vi "PLC Struct Byte Stream to G Object.vi"(8 "error in (no error)":errorcluster, 9 "[Sub-Item Type Information]":T1[](array[typedef]), 10 "Byte Stream":u8[](array[numeric]), 11 "TwinCAT ADS in":refnum<class "TwinCAT ADS.lvclass">) -> (0 "error out":errorcluster, 2 "Value":variant, 3 "TwinCAT ADS out":refnum<class "TwinCAT ADS.lvclass">)   [LabVIEW 2018, in "TwinCAT ADS.lvclass"]
uses:
  TwinCAT ADS.lvclass
  Controls/PLC Sub-Item Type Descriptor.ctl
  Controls/PLC Type.ctl
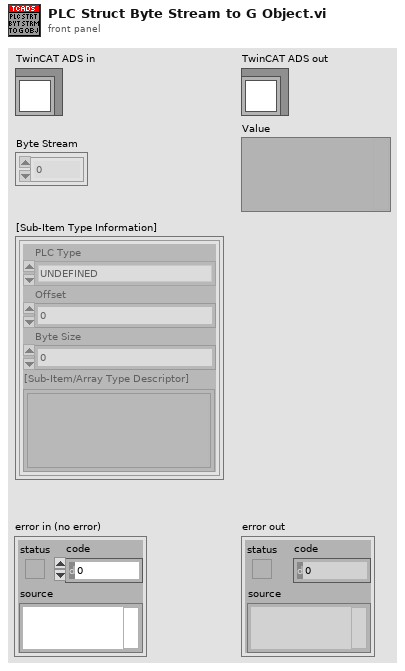
[diagram p1: front panel]
types:
  T1 = typedef "TwinCAT ADS.lvclass/PLC Sub-Item Type Descriptor.ctl" = cluster{"PLC Type":T2, "Offset":i32, "Byte Size":i32, "[Sub-Item/Array Type Descriptor]":variant[]}
  T2 = typedef "TwinCAT ADS.lvclass/PLC Type.ctl" = enum16{"UNDEFINED", "INT", "DINT", "REAL", "LREAL", "SINT", "BYTE", "UINT", "UDINT", "LINT", "ULINT", "STRING", "WSTRING", "BOOL", "TIME", "LTIME", "DATE", "DT", "TOD", "ARRAY", "JAGGED ARRAY", "STRUCT", "FUNCTION BLOCK", "UNION", "POINTER", "USER DEFINED"}
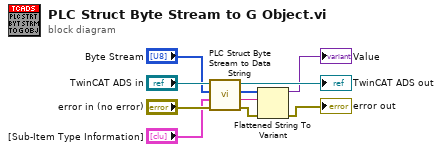
[diagram p0: block diagram]
diagram:
  n1 = call "PLC Struct Byte Stream to Data String.vi"("error in (no error)"="error in (no error)", "[Sub-Item Type Information]"="[Sub-Item Type Information]", "Byte Stream"="Byte Stream", "TwinCAT ADS in"="TwinCAT ADS in") -> ("error out"=w4:errorcluster, "Data String"=w3:string, "Type Descriptor"=w2:i16[], "TwinCAT ADS out"=→"TwinCAT ADS out":refnum<class "TwinCAT ADS.lvclass">)  [unwired: 4 in]
  n2 = Flattened String To Variant(4:w4, 6:w3, 7:w2) -> (0:→"error out":errorcluster, 3:→"Value":variant)
